vi "process.vi"(8 "error in (no error)":errorcluster, 10 "input":sgl[][](array[numeric]), 11 "GenericTraceProcessor in":refnum<class "GenericTraceProcessor.lvclass">) -> (0 "error out":errorcluster, 2 "output":sgl[][](array[numeric]), 3 "GenericTraceProcessor out":refnum<class "GenericTraceProcessor.lvclass">)   [LabVIEW 2010, in "GenericTraceProcessor.lvclass"]
uses:
  GenericTraceProcessor.lvclass
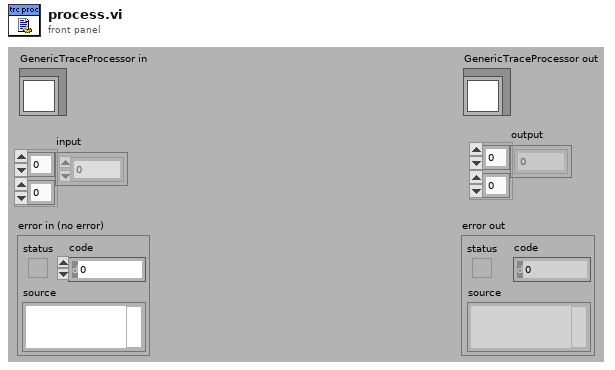
[diagram p1: front panel]
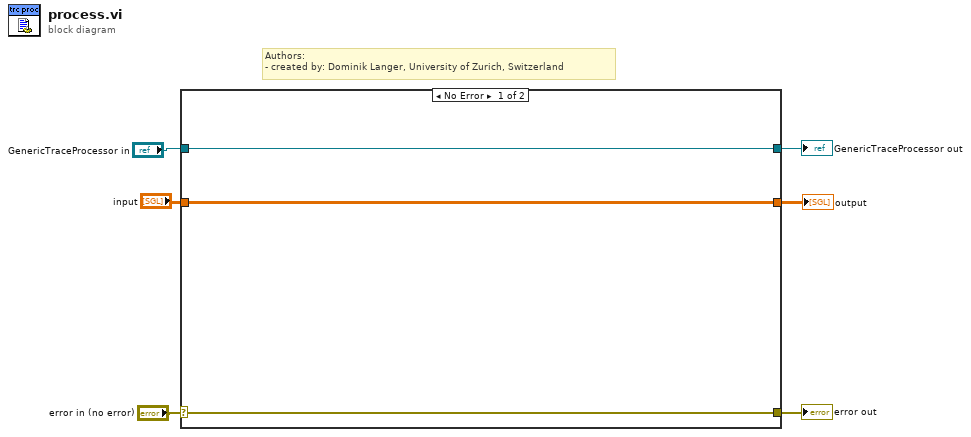
[diagram p0: block diagram]
diagram:
  # "Authors: \n- created by: Dominik Langer, University of Zurich, Switzerland"
  n1 = case shown="No Error" "error in (no error)" {
    selector: "error in (no error)" -> [w8 w12]
    tunnel: [w8 w12] -> w5
    tunnel: [w9 w11] -> w3
    tunnel: "GenericTraceProcessor in" -> [w9 w11]
    tunnel: "input" -> [w7 w10]
    tunnel: [w7 w10] -> w1
    frame No Error {
    }
    frame Error {
    }
  }
  "error out" <- w5
  "GenericTraceProcessor out" <- w3
  "output" <- w1
